vi "FTW-JSON-Validate.vi"(0 "JSON Opject":string, 11 "error in":errorcluster) -> (15 "error out":errorcluster)   [LabVIEW 2013]
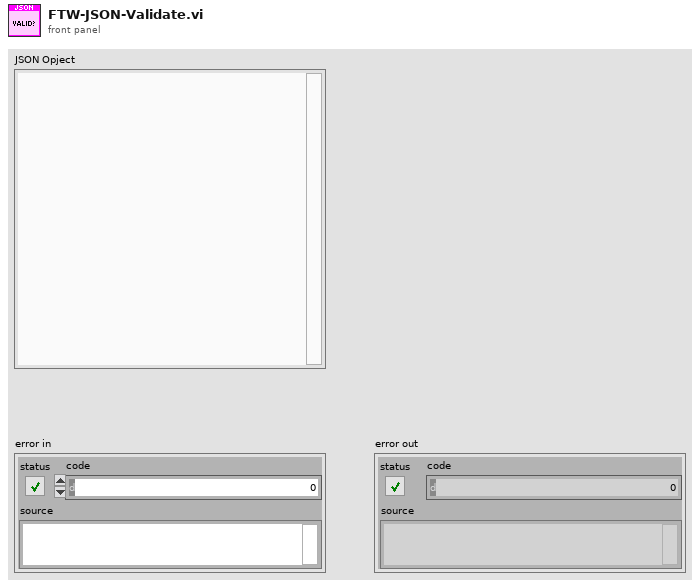
[diagram p1: front panel]
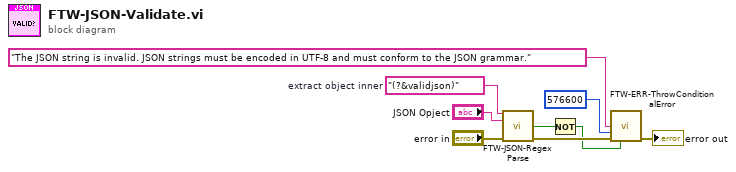
[diagram p0: block diagram]
diagram:
  w6 = "(?&validjson)"  # extract object inner
  n1 = call "FTW-JSON-RegexParse.vi"("Regular Expression using JSON subroutines"=w6, "Input String"="JSON Opject", "error in"="error in") -> ("Found Match?"=w2:bool, "error out"=w8:errorcluster)  [unwired: 8 in, 3 out]
  n2 = Not(x=w2) -> (.not. x?=w1:bool)
  n3 = call "FTW-ERR-ThrowConditionalError.vi"("Error Message"="The JSON string is invalid. JSON strings must be encoded in UTF-8 and must conform to the JSON grammar.", "Error Code"=576600, "error in"=w8, "Throw Error?"=w1) -> ("error out"=→"error out":errorcluster)  [unwired: 11 in]
